vi "Demo.vi"   [LabVIEW 2021, in "Ring Buffer Strict Accessor.lvlib"]
uses:
  Ring Buffer Strict Accessor.lvlib
  bb00c284-e980-43d4-ac83-bef45306a89d.vi
  c1ef7b93-11c8-4894-b2bf-59c5b04103fb.vi
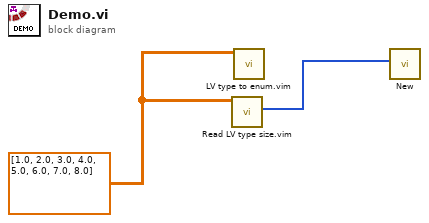
[diagram p0: block diagram]
diagram:
  w2 = dbl[][] [[1.0, 2.0, 3.0, 4.0], [5.0, 6.0, 7.0, 8.0]] ("LV type")
  n1 = call "Read LV type size.vim"("LV type"=w2) -> ("Size(s)"=w1:i32[])  [unwired: 9 in, 1 out]
  n2 = call "LV type to enum.vim"("LV Type"=w2) -> ()  [unwired: 8 in, 3 out]
  n3 = call "New.vi"("Size(s)"=w1) -> ()  [unwired: 9 in, 2 out]
